vi "fake_read.vi"(1 "line counter":u16, 2 "x resolution (pixels)":u16, 3 "y resolution (nr. of lines)":u16, 4 "Numeric":u64) -> (0 "input cluster":T1)   [LabVIEW 2010]
uses:
  common_typedefs/channels_cluster.ctl
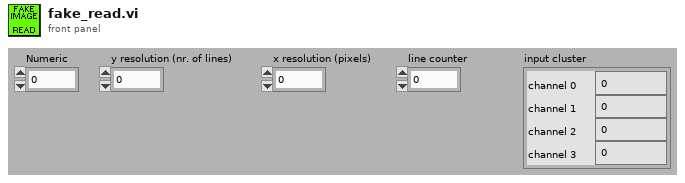
[diagram p1: front panel]
types:
  T1 = typedef "channels_cluster.ctl" = cluster{"channel 0":u32, "channel 1":u32, "channel 2":u32, "channel 3":u32}
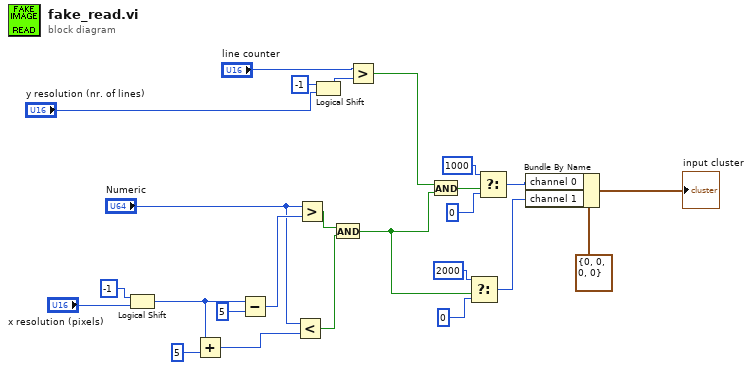
[diagram p0: block diagram]
diagram:
  n1 = Logical Shift(y=i16 -1 ("n"), x="x resolution (pixels)") -> (x << y=w9:u16)
  n2 = Add(x=w9, y=u16 5) -> (x+y=w3:u16)
  n3 = Subtract(x=w9, y=u16 5) -> (x-y=w6:u16)
  n4 = Less?(x="Numeric", y=w3) -> (x < y?=w2:bool)
  n5 = Greater?(x="Numeric", y=w6) -> (0:w5:bool)
  n6 = Logical Shift(y=i16 -1 ("n"), x="y resolution (nr. of lines)") -> (x << y=w13:u16)
  n7 = And(x=w5, y=w2) -> (x .and. y?=w1:bool)
  n8 = Greater?(x="line counter", y=w13) -> (0:w12:bool)
  n9 = And(x=w12, y=w1) -> (x .and. y?=w20:bool)
  n10 = Select(t=u16 2000 ("y"), s=w1, f=u16 0) -> (s? t:f=w16:u16)
  n11 = Select(t=u16 1000 ("y"), s=w20, f=u16 0) -> (s? t:f=w23:u16)
  n12 = Bundle By Name(cluster=T1 {"channel 0"=0, "channel 1"=0, "channel 2"=0, "channel 3"=0} ("input cluster"), "channel 0"=w23, "channel 1"=w16) -> (→"input cluster":T1)
